vi "FGV Map Set Data.vi"(8 "error in (no error)":errorcluster, 9 "Data In":variant, 10 "Data Key":string, 11 "Instance Key":string) -> (0 "error out":errorcluster, 2 "Instance Created ?":bool, 3 "Data Overwritten ?":bool)   [LabVIEW 2020, in "FGV Map.lvlib"]
uses:
  FGV Map.lvlib
  Controls/FGV Map Core State.ctl
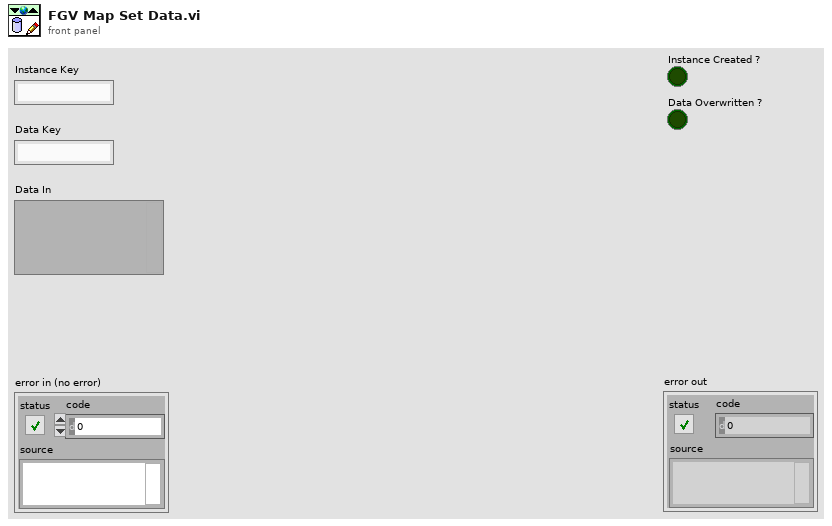
[diagram p1: front panel]
types:
  T1 = typedef "FGV Map.lvlib/FGV Map Core State.ctl" = enum16{"Init", "Set Instance (Unlock)", "Get Instance", "Get Instance (Lock)", "Unlock", "Get All Instances", "Delete Instance"}
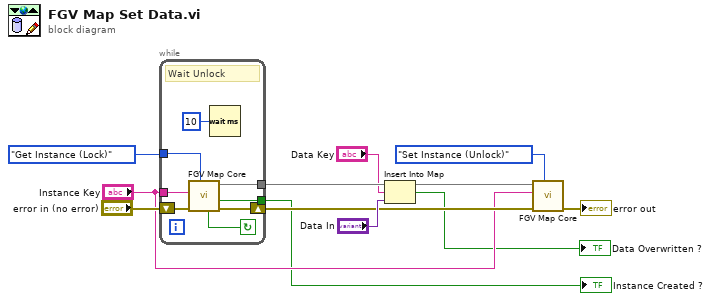
[diagram p0: block diagram]
diagram:
  n1 = while {
    tunnel: FGV_Map_Core_State."Get Instance (Lock)" ("FGV State") -> [w19]
    tunnel: [w18] -> w10
    tunnel: "Instance Key" -> [w16]
    shift-right: [w17] -> w6
    shift-left: "error in (no error)" -> [w20]
    tunnel: [w13] -> w1
    stop <- w15 continue-if-true
    # "Wait Unlock"
    n2 = call "FGV Map Core.vi"("FGV State"=w19, "error in"=w20, "Instance Key"=w16) -> ("error out"=w17:errorcluster, "Instance Not Found ?"=w13:bool, "Instance Out"=w18:map{string, variant}, "Was Locked ?"=w15:bool)  [unwired: 4 in, 1 out]
    n3 = Wait (ms)(milliseconds to wait=u32 10) -> ()  [unwired: 1 out]
  }
  "Instance Created ?" <- w1
  n4 = Insert Into Map(map in=w10, key="Data Key", value="Data In") -> (map out=w7:map{string, variant}, key already included?=→"Data Overwritten ?":bool)  [unwired: 1 out]
  n5 = call "FGV Map Core.vi"("FGV State"=FGV_Map_Core_State."Set Instance (Unlock)", "error in"=w6, "Instance Key"="Instance Key", "Instance In"=w7) -> ("error out"=→"error out":errorcluster)  [unwired: 3 in, 4 out]
